vi "CANShark_DeviceRead.vi"(10 "Timeout":i32, 11 "Device Handler":i64) -> (2 "CAN_Frame":u8[](array[numeric]), 3 "RX Return Value":i32)   [LabVIEW 2026]
uses:
  x64/Release/CanSharkApi_Dll1.dll
panel:
  out "error out":errorcluster
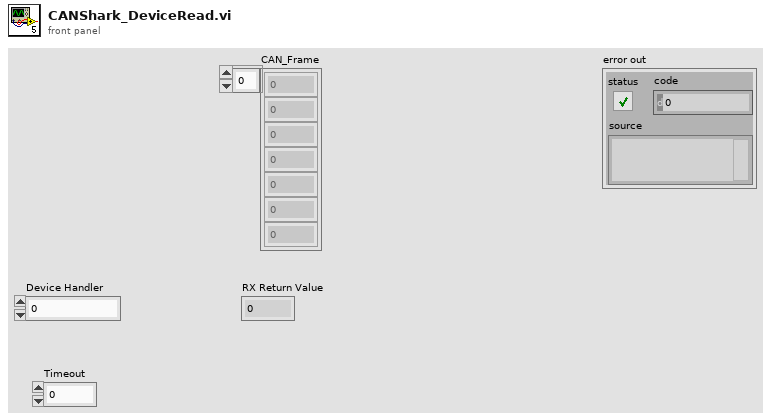
[diagram p1: front panel]
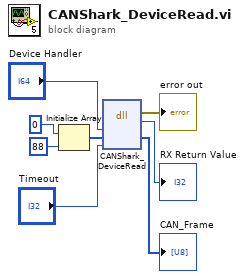
[diagram p0: block diagram]
diagram:
  n1 = Initialize Array(u8 0, u32 88) -> (w4:u8[])
  n2 = dll-call lib="C:/Users/TECQNIO/Documents/CANSHARK LABVIEW API PACKAGE/x64/Release/CanSharkApi_Dll1.dll" fn="CANShark_DeviceRead"("Device"="Device Handler", "CAN_Frame"=w4, "timeout"="Timeout") -> (error out=→"error out":errorcluster, "return type"=→"RX Return Value":i32, "CAN_Frame"=→"CAN_Frame":u8[])  [unwired: 5 in, 1 out]
